vi "AssertMultiChannelLoopbackForFixtureT-801.vi"(4 "DO Values":dbl[](array[numeric]), 5 "Tolerance":dbl=0.01 format="%#_13g", 6 "AO Values":dbl[](array[numeric]), 7 "Delay Time (s)":dbl=0.1 format="%#_13g", 8 "error in (no error)":errorcluster, 9 "Map from DO Master to DI Slave":map{string, string}(c390), 10 "Map from AO Master to AI Slave":map{string, string[]}(c390), 11 "VeriStand Test Case in":refnum<class "VeriStandTestCase.lvclass">) -> (0 "error out":errorcluster, 3 "VeriStand Test Case out":refnum<class "VeriStandTestCase.lvclass">)   [LabVIEW 2020, in "VeriStandTestCase.lvclass"]
uses:
  VeriStandTestCase.lvclass
  VeriStandTestCase.lvclass/VeriStandTestCase.ctl
  <vilib>/NI VeriStand/Execution/Workspace/NI VeriStand - Set Multiple Channel Values.vi
  <vilib>/NI VeriStand/Execution/Workspace/NI VeriStand - Get Multiple Channel Values.vi
  <vilib>/NI VeriStand/Execution/Workspace/NI_VS Workspace ExecutionAPI.lvlib
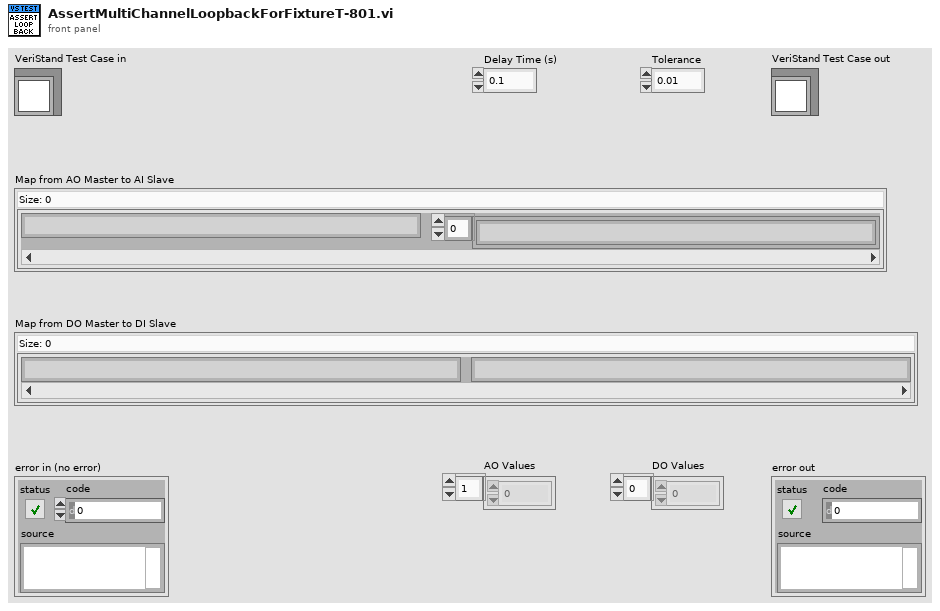
[diagram p1: front panel]
types:
  T1 = typedef "NI_VS Workspace ExecutionAPI.lvlib/WorkspaceAPI.ctl" = refnum<k24>
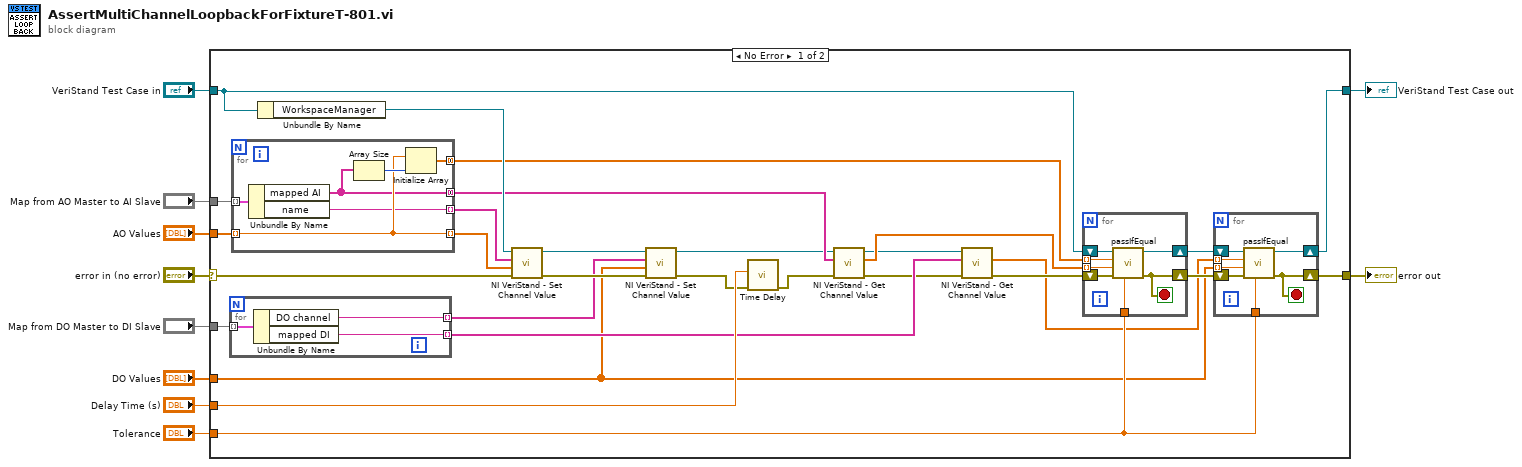
[diagram p0: block diagram]
diagram:
  n1 = case shown="No Error" "error in (no error)" {
    selector: "error in (no error)" -> [w39 w63]
    tunnel: [w14 w63] -> w10
    tunnel: "Map from DO Master to DI Slave" -> [w27 _]
    tunnel: "Map from AO Master to AI Slave" -> [w34 _]
    tunnel: "AO Values" -> [w31 _]
    tunnel: "Delay Time (s)" -> [w37 _]
    tunnel: "Tolerance" -> [w17 _]
    tunnel: "VeriStand Test Case in" -> [w36 w64]
    tunnel: [w13 w64] -> w5
    tunnel: "DO Values" -> [w11 _]
    frame No Error {
      n2 = for {
        tunnel: w27 -> [w49] mode=indexing
        tunnel: [w48] -> w24 mode=indexing
        tunnel: [w47] -> w21 mode=indexing
        n3 = Unbundle By Name(w49) -> ("DO channel"=w48:string, "mapped DI"=w47:string)
      }
      n4 = for {
        tunnel: w34 -> [w55] mode=indexing
        tunnel: [w50] -> w33 mode=indexing
        tunnel: [w53] -> w32 mode=indexing
        tunnel: w31 -> [w53] mode=indexing
        tunnel: [w52] -> w30 mode=concatenating
        tunnel: [w51] -> w28 mode=concatenating
        n5 = Unbundle By Name(w55) -> ("mapped AI"=w51:string[], "name"=w50:string)
        n6 = Array Size(array=w51) -> (size(s)=w54:i32)
        n7 = Initialize Array(w53, w54) -> (w52:dbl[])
      }
      n8 = Unbundle By Name(w36) -> ("WorkspaceManager"=w35:T1)
      n9 = call-poly <vilib>:"NI VeriStand - Set Channel Value.vi"("error in (no error)"=w39, "Values"=w32, "Channels"=w33, "WorkspaceManager in"=w35) -> ("error out"=w25:errorcluster, "WorkspaceManager out"=w26:T1)  [unwired: 6 in]
      n10 = call-poly <vilib>:"NI VeriStand - Set Channel Value.vi"("error in (no error)"=w25, "Values"=w11, "Channels"=w24, "WorkspaceManager in"=w26) -> ("error out"=w22:errorcluster, "WorkspaceManager out"=w23:T1)  [unwired: 6 in]
      n11 = call "Time Delay"("error in (no error)"=w22, "Delay Time (s)"=w37) -> ("error out"=w38:errorcluster)  [unwired: 9 in]
      n12 = call-poly <vilib>:"NI VeriStand - Get Channel Value.vi"("error in (no error)"=w38, "Channels"=w28, "WorkspaceManager in"=w23) -> ("error out"=w19:errorcluster, "Values"=w29:dbl[], "WorkspaceManager out"=w20:T1)  [unwired: 6 in]
      n13 = call-poly <vilib>:"NI VeriStand - Get Channel Value.vi"("error in (no error)"=w19, "Channels"=w21, "WorkspaceManager in"=w20) -> ("error out"=w18:errorcluster, "Values"=w12:dbl[])  [unwired: 6 in, 1 out]
      n14 = for {
        tunnel: w17 -> [w61]
        shift-right: [w58] -> w15
        shift-left: w18 -> [w62]
        shift-right: [w60] -> w16
        shift-left: w36 -> [w59]
        tunnel: w30 -> [w57] mode=indexing
        tunnel: w29 -> [w56] mode=indexing
        stop <- w58 stop-if-true
        n15 = call-dynamic "passIfEqual.vi"("delta (optional)"=w61, "error in (no error)"=w62, "y"=w56, "x"=w57, "TestCase in"=w59) -> ("error out"=w58:errorcluster, "TestCase out"=w60:refnum<class "VeriStandTestCase.lvclass">)  [unwired: 5 in]
      }
      n16 = for {
        tunnel: w17 -> [w45]
        shift-right: [w42] -> w14
        shift-left: w15 -> [w46]
        shift-right: [w44] -> w13
        shift-left: w16 -> [w43]
        tunnel: w12 -> [w41] mode=indexing
        tunnel: w11 -> [w40] mode=indexing
        stop <- w42 stop-if-true
        n17 = call-dynamic "passIfEqual.vi"("delta (optional)"=w45, "error in (no error)"=w46, "y"=w40, "x"=w41, "TestCase in"=w43) -> ("error out"=w42:errorcluster, "TestCase out"=w44:refnum<class "VeriStandTestCase.lvclass">)  [unwired: 5 in]
      }
    }
    frame Error {
    }
  }
  "error out" <- w10
  "VeriStand Test Case out" <- w5
